vi "Raft_wars_Ver4.vi"() -> ()   [LabVIEW 2026]
panel:
  out "x .and. y?":bool
  out "x .or. y?":bool
  out "Array":dbl[][](array[numeric])
  in  "Player Ship Inputs":T1(array[cluster]) {"Y-Coordinate" min=0 max=7; "X-Coordinate" min=0 max=7}
  in  "Emergency Stop":bool
  out "Game Status":string
  out "Ships Placed":dbl
  out "Losses":dbl
  out "Computer Hits":dbl
  out "Wins":dbl
  out "Player Hits":dbl
  in  "Attack":bool
  in  "Play Again":bool
  in  "Place Ship":bool
  in  "Attack Y":dbl
  in  "Attack X":dbl
  in  "Ship Y":i32
  in  "Ship X":i32
  out "Computer  Board":u32[][][][][][][][](array[colorbox])
  out "Player Board":u32[][][][][][][][](array[colorbox])
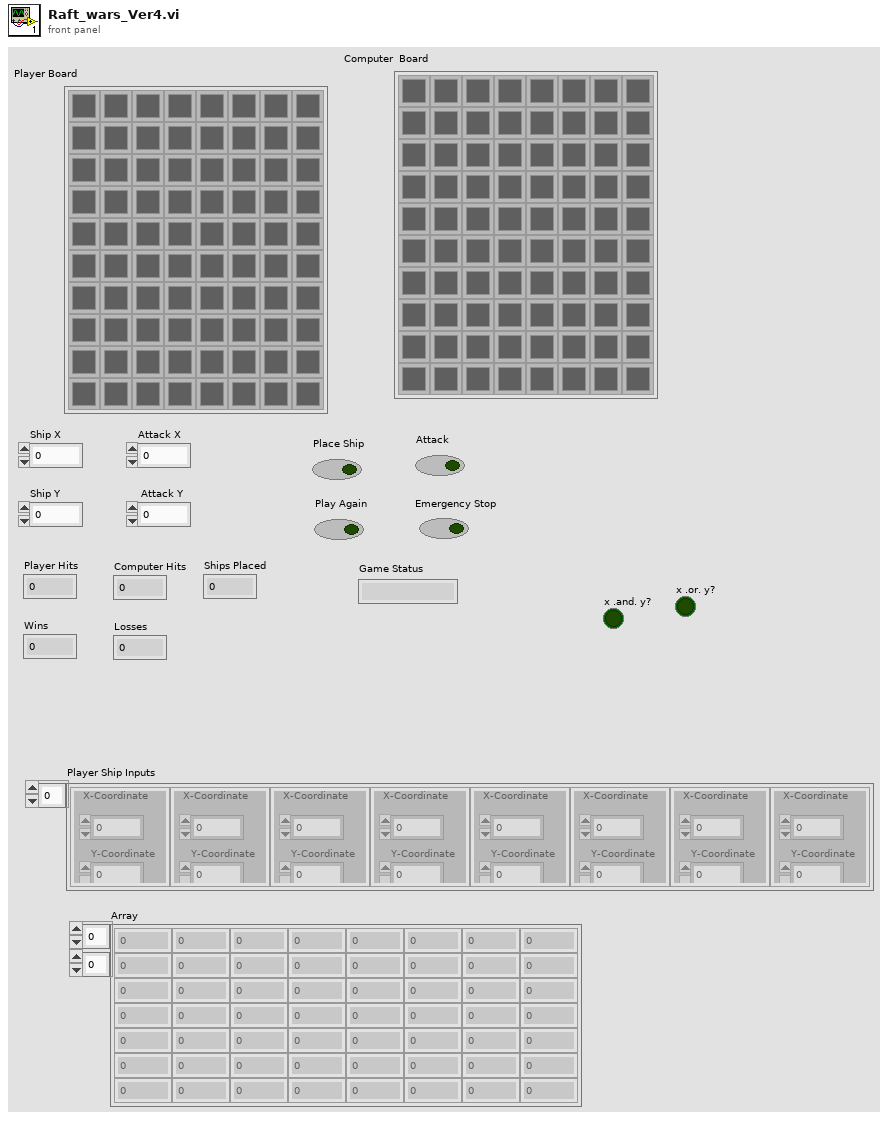
[diagram p1: front panel]
types:
  T1 = cluster{"X-Coordinate":i32, "Y-Coordinate":i32}[]
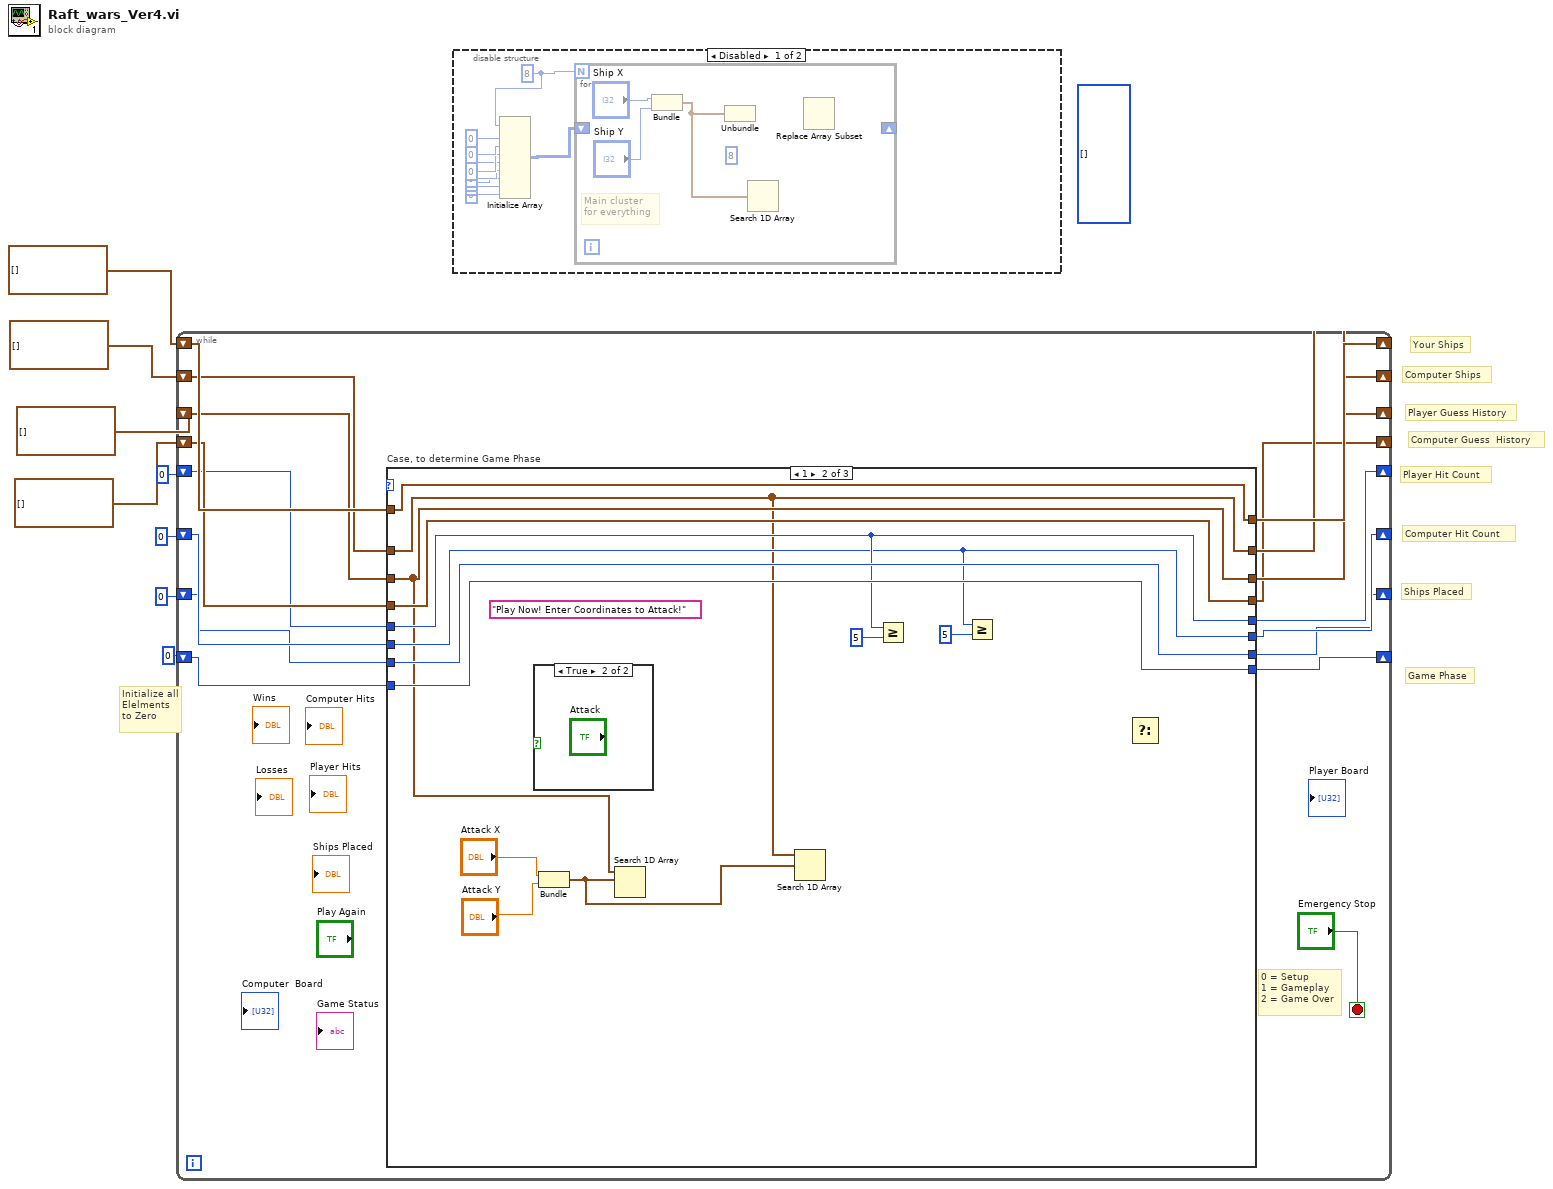
[diagram p0: block diagram]
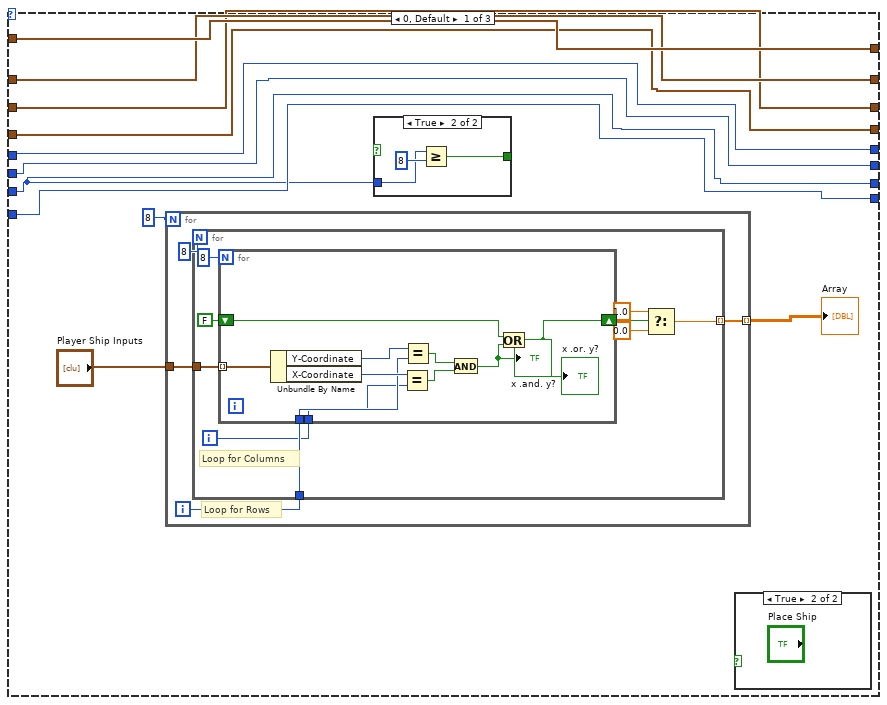
[diagram p3: hidden frame]
diagram:
  (unwired) u32[][][][][][][][] [] ("PLayer 1 Board 2")
  # "Initialize all\nElelments\nto Zero"
  # "Ships Placed"
  # "Your Ships"
  # "Computer Ships"
  # "Player Guess History"
  # "Computer Guess  History"
  # "Player Hit Count"
  # "Computer Hit Count"
  # "Game Phase"
  n1 = while {
    shift-right: [w23] -> _
    shift-left: cluster{dbl, dbl}[] [] -> [w24]
    shift-right: [w21] -> _
    shift-left: cluster{dbl, dbl}[] [] -> [w22]
    shift-right: [w19] -> _
    shift-left: cluster{dbl, dbl}[] [] -> [w20]
    shift-right: [w17] -> _
    shift-left: cluster{dbl, dbl}[] [] -> [w18]
    shift-right: [w12] -> _
    shift-left: 0 -> [w16]
    shift-right: [w11] -> _
    shift-left: 0 -> [w15]
    shift-right: [w10] -> _
    shift-left: 0 -> [w14]
    shift-right: [w9] -> _
    shift-left: 0 -> [w13]
    stop <- "Emergency Stop" stop-if-true
    # "0 = Setup\n1 = Gameplay\n2 = Game Over"
    n2 = case "Case, to determine Game Phase" shown="1" {
      selector: _ -> [_ _ _]
      tunnel: w24 -> [w36 w75 w83]
      tunnel: [w36 w75 w83] -> w23
      tunnel: w22 -> [w35 w64 w82]
      tunnel: [w35 w64 w82] -> w21
      tunnel: w20 -> [w34 w65 w81]
      tunnel: [w34 w65 w81] -> w19
      tunnel: w18 -> [w33 w74 w80]
      tunnel: [w33 w74 w80] -> w17
      tunnel: w16 -> [w29 w70 w79]
      tunnel: w15 -> [w28 w68 w78]
      tunnel: w14 -> [w26 w73 w77]
      tunnel: w13 -> [w27 w72 w76]
      tunnel: [w29 w70 w79] -> w12
      tunnel: [w28 w68 w78] -> w11
      tunnel: [w26 w73 w77] -> w10
      tunnel: [w27 w72 w76] -> w9
      frame 0, Default {
        n3 = for {
          N: 8 -> [_]
          tunnel: "Player Ship Inputs" -> [w40]
          tunnel: [w41] -> w32 mode=indexing
          i -> [w42]
          # "Loop for Rows"
          n4 = for {
            N: 8 -> [_]
            tunnel: w42 -> [w52]
            tunnel: [w47] -> w41 mode=indexing
            tunnel: w40 -> [w44]
            i -> [w51]
            # "Loop for Columns"
            n5 = for {
              N: 8 -> [_]
              tunnel: w52 -> [w55]
              tunnel: w51 -> [w54]
              shift-right: [w56] -> w50
              shift-left: FALSE -> [w57]
              tunnel: w44 -> [w53] mode=indexing
              n6 = Unbundle By Name(w53) -> ("Y-Coordinate"=w61:i32, "X-Coordinate"=w62:i32)
              n7 = Equal?(x=w62, y=w54) -> (x = y?=w59:bool)
              n8 = Equal?(x=w61, y=w55) -> (x = y?=w60:bool)
              n9 = And(x=w60, y=w59) -> (x .and. y?=w58:bool)
              "x .and. y?" <- w58
              n10 = Or(x=w57, y=w58) -> (x .or. y?=w56:bool)
              "x .or. y?" <- w56
            }
            n11 = Select(t=1.0, s=w50, f=0.0) -> (s? t:f=w47:dbl)
          }
        }
        "Array" <- w32
        n12 = case shown="True" {
          selector: _ -> [_ _]
          tunnel: w26 -> [_ w38]
          tunnel: [_ w37] -> _
          frame False {
          }
          frame True {
            n13 = Greater Or Equal?(x=w38, y=8) -> (x >= y?=w37:bool)
          }
        }
        n14 = case shown="True" {
          selector: _ -> [_ _]
          frame False {
          }
          frame True {
          }
        }
      }
      frame 1 {
        (unwired) "Play Now! Enter Coordinates to Attack!"
        n15 = case shown="True" {
          selector: _ -> [_ _]
          frame False {
          }
          frame True {
          }
        }
        n16 = Bundle("Attack X"="Attack X", "Attack Y"="Attack Y") -> (w63:cluster{"Attack X":dbl, " Attack Y":dbl})  [unwired: 1 in]
        n17 = Search 1D Array(1D array=w65, element=w63) -> ()  [unwired: 1 in, 1 out]
        n18 = Search 1D Array(1D array=w64, element=w63) -> ()  [unwired: 1 in, 1 out]
        n19 = Greater Or Equal?(x=w70, y=5) -> ()  [unwired: 1 out]
        n20 = Greater Or Equal?(x=w68, y=5) -> ()  [unwired: 1 out]
        n21 = Select() -> ()  [unwired: 3 in, 1 out]
      }
      frame 2 {
      }
    }
  }
  n22 = disable-structure shown="Disabled" {
    frame Disabled {
      w92 = 8
      n23 = Initialize Array(w92, 0 ("dimension size"), 0 ("dimension size"), 0 ("dimension size"), 0 ("dimension size"), 0 ("dimension size"), 0 ("dimension size"), 0 ("dimension size"), 0 ("dimension size")) -> (w93:i32[][][][][][][][])
      n24 = for {
        N: w92 -> [_]
        shift-right: _ -> [w94]
        shift-left: w93 -> [_]
        (unwired) 8
        # "Main cluster\nfor everything"
        n25 = Bundle("Ship X"="Ship X", "Ship Y"="Ship Y") -> (w95:cluster{"Ship X":i32, "Ship Y":i32})  [unwired: 1 in]
        n26 = Unbundle(w95) -> ()  [unwired: 2 out]
        n27 = Search 1D Array(element=w95) -> ()  [unwired: 2 in, 1 out]
        n28 = Replace Array Subset() -> ()  [unwired: 3 in, 1 out]
      }
    }
    frame Enabled {
    }
  }
